vi "Get Result.vi"(4 "Controller name":string, 6 "Last request":bool, 8 "error in (no error)":errorcluster, 11 "Instrument Recorder in":refnum<class "DataSocket Client.lvclass">) -> (0 "error out":errorcluster, 2 "Result":refnum<class "Acquired Result.lvclass">, 3 "Instrument Recorder out":refnum<class "DataSocket Client.lvclass">)   [LabVIEW 2021, in "DataSocket Client.lvclass"]
uses:
  DataSocket Client.lvclass
  DataSocket Client.lvclass/DataSocket Client.ctl
  NHMFL_Core/Libraries/Instruments/Results/Acquired Result/Acquired Result.lvclass
  <vilib>/express/express signal manip/GetorSetDDTAttributes/Set DDT Attributes/Set DDT Properties.xnode
  <vilib>/express/express shared/transition.llb/Dynamic To Waveform Array.vi
  <vilib>/express/express signal manip/GetorSetDDTAttributes/Set DDT Attributes/SetT0.vi
  <vilib>/express/express shared/transition.llb/Waveform Array To Dynamic.vi
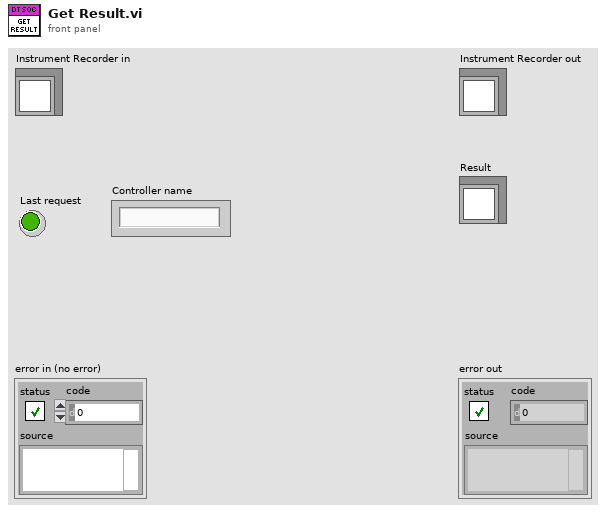
[diagram p1: front panel]
types:
  T1 = typedef "DataSocket Configuration.ctl" = cluster{"DataSocket  URLs":string[]}
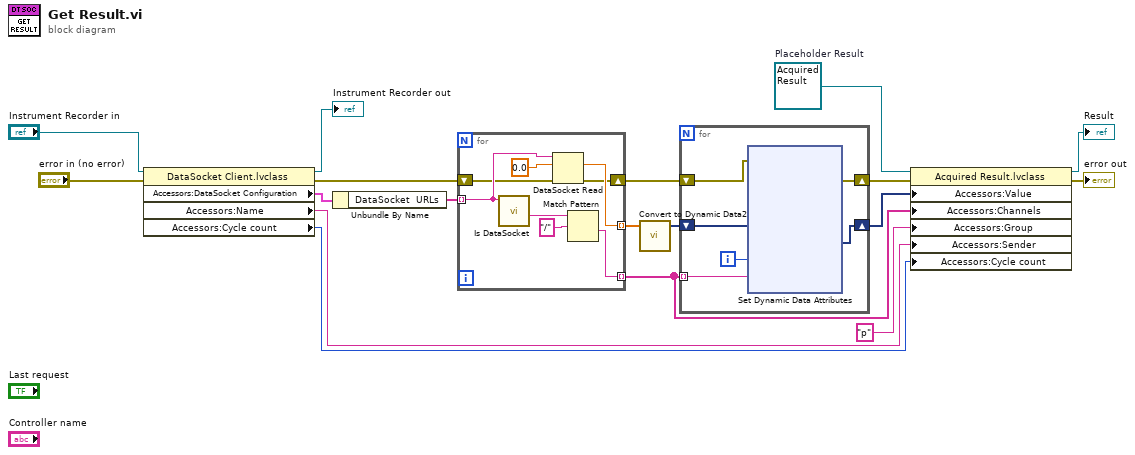
[diagram p0: block diagram]
diagram:
  w9 = refnum<class "Acquired Result.lvclass"> refnum  # Placeholder Result
  n1 = property class="DataSocket Client.lvclass"(reference="Instrument Recorder in", error in="error in (no error)") -> (reference out=→"Instrument Recorder out":refnum<class "DataSocket Client.lvclass">, error out=w6:errorcluster, "Accessors:DataSocket Configuration"=w17:T1, "Accessors:Name"=w10:string, "Accessors:Cycle count"=w1:i32)
  n2 = Unbundle By Name(w17) -> ("DataSocket  URLs"=w16:string[])
  n3 = for {
    tunnel: w16 -> [w25] mode=indexing
    tunnel: [w22] -> w12 mode=indexing
    tunnel: [w21] -> w15 mode=indexing
    shift-right: [w20] -> w7
    shift-left: w6 -> [w19]
    n4 = call "Is DataSocket.vi"("String"=w25) -> ("After header"=w24:string)  [unwired: 9 in, 1 out]
    n5 = DataSocket Read(8:w19, 10:0.0 ("DBL Value"), 11:w25) -> (0:w20:errorcluster, 2:w21:dbl)  [unwired: 2 in, 5 out]
    n6 = Match Pattern(string=w24, regular expression="/") -> (after substring=w22:string)  [unwired: 1 in, 3 out]
  }
  n7 = call "Convert to Dynamic Data2"("Array"=w15) -> ("Dynamic Data Type"=w14:dynamicdata)  [unwired: 3 in]
  n8 = for {
    tunnel: w12 -> [w29] mode=indexing
    shift-right: [w31] -> w13
    shift-left: w14 -> [w32]
    shift-right: [w28] -> w8
    shift-left: w7 -> [w27]
    i -> [w30]
    n9 = xnode "Set Dynamic Data Attributes"("Signals In"=w32, "Signal Index"=w30, "Signal Name"=w29, "error in"=w27) -> ("Signals Out"=w31:dynamicdata, "error out"=w28:errorcluster)
  }
  n10 = property class="Acquired Result.lvclass"(reference=w9, error in=w8, "Accessors:Value"=w13, "Accessors:Channels"=w12, "Accessors:Group"="p" ("Group"), "Accessors:Sender"=w10, "Accessors:Cycle count"=w1) -> (reference out=→"Result":refnum<class "Acquired Result.lvclass">, error out=→"error out":errorcluster)
